vi "Matrix Inverse v1.1.vi"() -> ()   [LabVIEW 2020]
uses:
  <vilib>/Analysis/Matrix/Datatypes/RealMatrix.ctl
  <vilib>/Analysis/Matrix/Numeric/Conversions/Array To Matrix - RA2.vi
  <vilib>/Analysis/baseanly.llb/Real Inverse Matrix.vi
  <vilib>/Analysis/Matrix/Numeric/Conversions/Matrix To Array - RM.vi
  <vilib>/Analysis/NI_AALBase.lvlib
  <vilib>/Analysis/Matrix/NI_Matrix.lvlib
panel:
  out "divide by zero detected":bool
  out "Joint Matrix":sgl[][](array[numeric])
  out "A":T1
  out "sum of error":sgl
  out "inv(A) LABVIEW-FPGA":sgl[][](array[numeric])
  out "inv(A) LABVIEW":T1
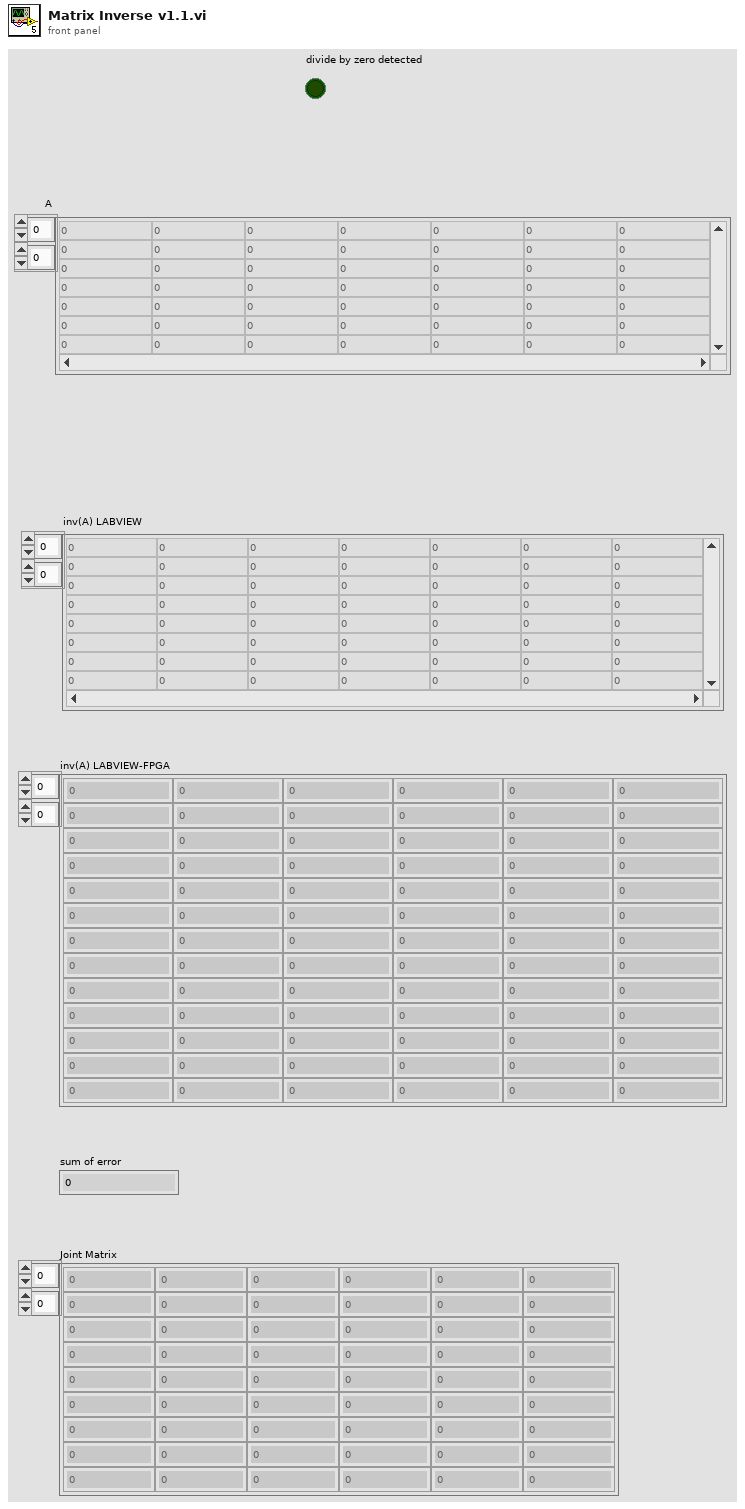
[diagram p1: front panel]
types:
  T1 = typedef "NI_Matrix.lvlib/RealMatrix.ctl" = dbl[][]
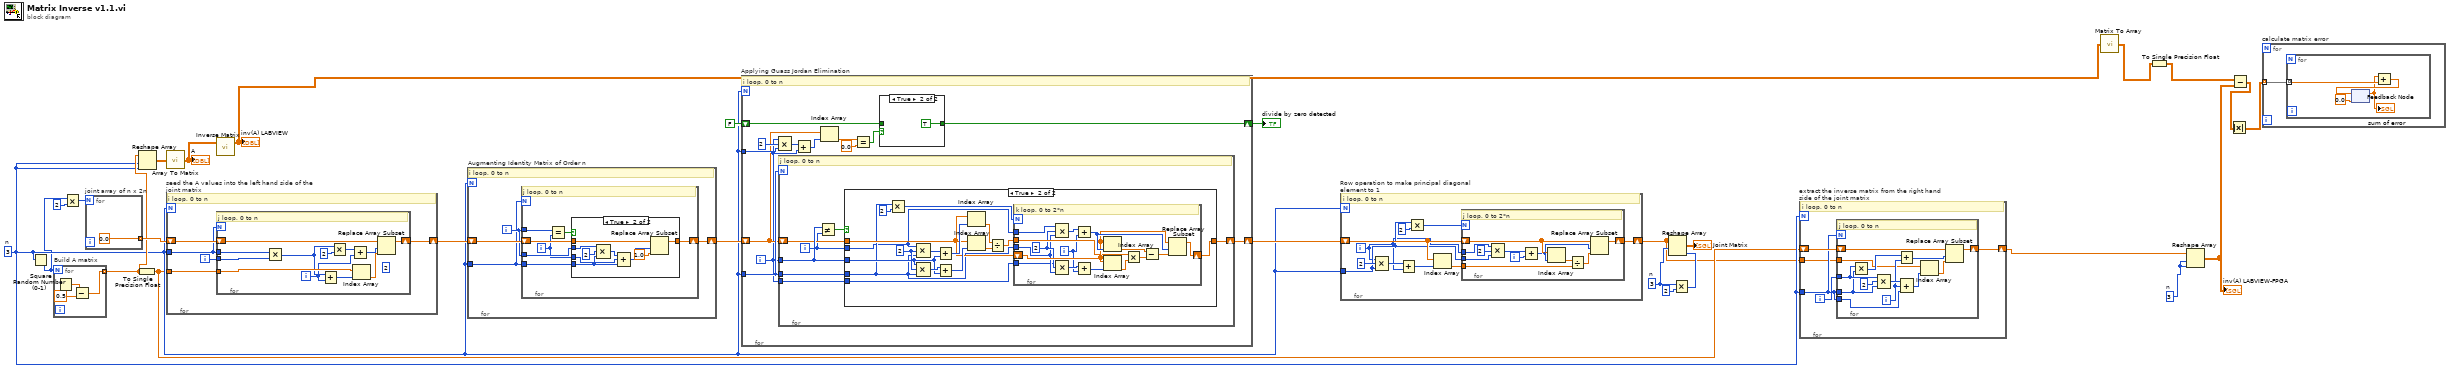
[diagram p0: block diagram]
diagram:
  w9 = 3  # n
  w24 = 3  # n
  w12 = 3  # n
  n1 = Square(x=w12) -> (x^2=w1:i32)
  n2 = for "Build A matrix" {
    N: w1 -> [_]
    tunnel: [w28] -> w13 mode=indexing
    n3 = Random Number (0-1)() -> (number: 0 to 1=w30:dbl)
    n4 = Subtract(x=w30, y=0.5) -> (x-y=w28:dbl)
  }
  n5 = Multiply(x=w1, y=2) -> (x*y=w20:i32)
  n6 = for "joint array of n x 2n" {
    N: w20 -> [_]
    tunnel: [sgl 0.0] -> w19 mode=indexing
  }
  n7 = Reshape Array(w13, w12, w12) -> (w27:dbl[][])
  n8 = To Single Precision Float(number=w13) -> (single precision float=w11:sgl[])
  n9 = call-poly <vilib>:"Array To Matrix.vi"("Real 2D Array"=w27) -> ("Real Matrix"=w26:T1)
  "A" <- w26
  n10 = for "seed the A values into the left hand side of the joint matrix" {
    N: w12 -> [_]
    shift-right: [w35] -> w18
    shift-left: w19 -> [w36]
    tunnel: w12 -> [w34]
    tunnel: w11 -> [w33]
    i -> [w32]
    # "i loop, 0 to n"
    n11 = for {
      N: w34 -> [_]
      shift-right: [w47] -> w35
      shift-left: w36 -> [w48]
      tunnel: w34 -> [w44]
      tunnel: w33 -> [w46]
      tunnel: w32 -> [w45]
      i -> [w38]
      (unwired) 2
      # "j loop, 0 to n"
      n12 = Multiply(x=w44, y=w45) -> (x*y=w40:i32)
      n13 = Add(x=w40, y=w38) -> (x+y=w43:i32)
      n14 = Multiply(x=w40, y=2) -> (x*y=w39:i32)
      n15 = Add(x=w39, y=w38) -> (x+y=w37:i32)
      n16 = Index Array(array=w46, index=w43) -> (element=w42:sgl)
      n17 = Replace Array Subset(array=w48, new element=w42, index=w37) -> (w47:sgl[])
    }
  }
  n18 = call-poly <vilib>:"Inverse Matrix.vi"("Input Matrix"=w26) -> ("Inverse Matrix"=w5:T1)  [unwired: 1 in, 1 out]
  "inv(A) LABVIEW" <- w5
  n19 = for "Augmenting Identity Matrix of Order n" {
    N: w12 -> [_]
    shift-right: [w51] -> w15
    shift-left: w18 -> [w52]
    tunnel: w12 -> [w49]
    i -> [w50]
    # "i loop, 0 to n"
    n20 = for {
      N: w49 -> [_]
      tunnel: w50 -> [w59]
      shift-right: [w56] -> w51
      shift-left: w52 -> [w57]
      tunnel: w50 -> [w55]
      tunnel: w49 -> [w54]
      i -> [w53]
      # "j loop, 0 to n"
      n21 = Equal?(x=w59, y=w53) -> (x = y?=w58:bool)
      n22 = case shown="True" w58 {
        tunnel: w57 -> [w60 w69]
        tunnel: [w60 w65] -> w56
        tunnel: w55 -> [_ w67]
        tunnel: w54 -> [_ w62]
        tunnel: w53 -> [_ w63]
        frame False {
        }
        frame True {
          n23 = Compound Arithmetic op=MULTIPLY(w67, 2, w62) -> (w64:i32)
          n24 = Compound Arithmetic op=ADD(w64, w63, w62) -> (w61:i32)
          n25 = Replace Array Subset(array=w69, new element=sgl 1.0 ("new element/subarray"), index=w61) -> (w65:sgl[])
        }
      }
    }
  }
  n26 = for "Applying Guass Jordan Elimination" {
    N: w12 -> [_]
    tunnel: w12 -> [w80]
    shift-right: [w74] -> w16
    shift-left: FALSE -> [w75]
    tunnel: w12 -> [w73]
    shift-right: [w70] -> w14
    shift-left: w15 -> [w72]
    i -> [w71]
    # "i loop, 0 to n"
    n27 = Compound Arithmetic op=MULTIPLY(w71, 2 ("value"), w80) -> (w79:i32)
    n28 = for {
      N: w73 -> [_]
      tunnel: w71 -> [w88]
      tunnel: w73 -> [w89]
      tunnel: w71 -> [w84]
      shift-right: [w83] -> w70
      shift-left: w72 -> [w87]
      i -> [w85]
      # "j loop, 0 to n"
      n29 = Not Equal?(x=w88, y=w85) -> (x != y?=w86:bool)
      n30 = case shown="True" w86 {
        tunnel: w89 -> [_ w95]
        tunnel: w88 -> [_ w97]
        tunnel: w87 -> [w90 w96]
        tunnel: w85 -> [_ w94]
        tunnel: w84 -> [_ w92]
        tunnel: [w90 w91] -> w83
        frame False {
        }
        frame True {
          w101 = 2 ("value")
          n31 = Multiply(x=w95, y=2 ("value")) -> (x*y=w98:i32)
          n32 = Compound Arithmetic op=MULTIPLY(w94, w101, w95) -> (w106:i32)
          n33 = Compound Arithmetic op=MULTIPLY(w97, w101, w95) -> (w102:i32)
          n34 = Add(x=w106, y=w97) -> (x+y=w105:i32)
          n35 = Add(x=w102, y=w97) -> (x+y=w100:i32)
          n36 = Index Array(array=w96, index=w105) -> (element=w104:sgl)
          n37 = Index Array(array=w96, index=w100) -> (element=w103:sgl)
          n38 = Divide(x=w104, y=w103) -> (x/y=w93:sgl)
          n39 = for {
            N: w98 -> [_]
            tunnel: w95 -> [w113]
            tunnel: w94 -> [w121]
            tunnel: w93 -> [w117]
            tunnel: w92 -> [w112]
            shift-right: [w107] -> w91
            shift-left: w96 -> [w119]
            i -> [w115]
            w114 = 2 ("value")
            # "k loop, 0 to 2*n"
            n40 = Compound Arithmetic op=MULTIPLY(w121, w114, w113) -> (w122:i32)
            n41 = Compound Arithmetic op=MULTIPLY(w112, w114, w113) -> (w116:i32)
            n42 = Add(x=w122, y=w115) -> (x+y=w120:i32)
            n43 = Add(x=w116, y=w115) -> (x+y=w111:i32)
            n44 = Index Array(array=w119, index=w120) -> (element=w109:sgl)
            n45 = Index Array(array=w119, index=w111) -> (element=w118:sgl)
            n46 = Multiply(x=w117, y=w118) -> (x*y=w110:sgl)
            n47 = Subtract(x=w109, y=w110) -> (x-y=w108:sgl)
            n48 = Replace Array Subset(array=w119, new element=w108, index=w120) -> (w107:sgl[])
          }
        }
      }
    }
    n49 = Add(x=w79, y=w71) -> (x+y=w78:i32)
    n50 = Index Array(array=w72, index=w78) -> (element=w77:sgl)
    n51 = Equal?(x=w77, y=sgl 0.0) -> (x = y?=w76:bool)
    n52 = case shown="True" w76 {
      tunnel: w75 -> [w123 _]
      tunnel: [w123 TRUE] -> w74
      frame False {
      }
      frame True {
      }
    }
  }
  "divide by zero detected" <- w16
  n53 = for "Row operation to make principal diagonal element to 1" {
    N: w12 -> [_]
    tunnel: w12 -> [w128]
    shift-right: [w125] -> w8
    shift-left: w14 -> [w129]
    i -> [w127]
    # "i loop, 0 to n"
    n54 = Compound Arithmetic op=MULTIPLY(w127, 2 ("value"), w128) -> (w133:i32)
    n55 = Add(x=w133, y=w127) -> (x+y=w132:i32)
    n56 = Multiply(x=w128, y=2) -> (x*y=w130:i32)
    n57 = Index Array(array=w129, index=w132) -> (element=w126:sgl)
    n58 = for {
      N: w130 -> [_]
      tunnel: w128 -> [w144]
      tunnel: w127 -> [w143]
      tunnel: w126 -> [w139]
      shift-right: [w137] -> w125
      shift-left: w129 -> [w138]
      i -> [w141]
      # "j loop, 0 to 2*n"
      n59 = Compound Arithmetic op=MULTIPLY(w143, 2 ("value"), w144) -> (w142:i32)
      n60 = Add(x=w142, y=w141) -> (x+y=w136:i32)
      n61 = Index Array(array=w138, index=w136) -> (element=w140:sgl)
      n62 = Divide(x=w140, y=w139) -> (x/y=w135:sgl)
      n63 = Replace Array Subset(array=w138, new element=w135, index=w136) -> (w137:sgl[])
    }
  }
  n64 = Multiply(x=w24, y=2) -> (x*y=w23:i32)
  n65 = Reshape Array(w8, w24, w23) -> (→"Joint Matrix":sgl[][])
  n66 = for "extract the inverse matrix from the right hand side of the joint matrix" {
    N: w12 -> [_]
    tunnel: w12 -> [w147]
    shift-right: [w149] -> w10
    shift-left: w11 -> [w150]
    tunnel: w8 -> [w146]
    i -> [w148]
    # "i loop, 0 to n"
    n67 = for {
      N: w147 -> [_]
      shift-right: [w162] -> w149
      shift-left: w150 -> [w163]
      tunnel: w148 -> [w159]
      tunnel: w147 -> [w157]
      tunnel: w147 -> [w154]
      tunnel: w146 -> [w152]
      i -> [w155]
      # "j loop, 0 to n"
      n68 = Multiply(x=w159, y=w157) -> (x*y=w161:i32)
      n69 = Compound Arithmetic op=MULTIPLY(w159, 2, w157) -> (w156:i32)
      n70 = Add(x=w161, y=w155) -> (x+y=w160:i32)
      n71 = Compound Arithmetic op=ADD(w156, w155, w154) -> (w153:i32)
      n72 = Index Array(array=w152, index=w153) -> (element=w151:sgl)
      n73 = Replace Array Subset(array=w163, new element=w151, index=w160) -> (w162:sgl[])
    }
  }
  n74 = call-poly <vilib>:"Matrix To Array.vi"("Real Matrix"=w5) -> ("Real 2D Array"=w3:dbl[][])
  n75 = To Single Precision Float(number=w3) -> (single precision float=w2:sgl[][])
  n76 = Reshape Array(w10, w9, w9) -> (w4:sgl[][])
  "inv(A) LABVIEW-FPGA" <- w4
  n77 = Subtract ("Subtract.vi")(x=w2, y=w4) -> (x-y=w7:sgl[][])
  n78 = Absolute Value ("Absolute Value.vi")(x=w7) -> (abs(x)=w6:sgl[][])
  n79 = for "calculate matrix error" {
    tunnel: w6 -> [w164] mode=indexing
    n80 = for {
      tunnel: w164 -> [w168] mode=indexing
      n81 = feedback #1(sgl 0.0) -> (w166:sgl)
      "sum of error" <- w166
      n82 = Add(x=w166, y=w168) -> (x+y=w167:sgl)
      n83 = feedback-in #1(w167) -> ()
    }
  }
